vi "Auto Execute Commands.vi"() -> ()   [LabVIEW 2019]
uses:
  Controls/Auto Controls.ctl
  <vilib>/Rock Robotics/WPI/Solenoid/WPI_SolenoidValue.ctl
  <vilib>/Rock Robotics/WPI/Solenoid/WPI_SolenoidSetEnum.vi
panel:
  in  "Auto Commands":T1=[{"Drive Duration"=0.0, "Left Speed"=0.0, "Right Speed"=0.0, "Set Point"=0.0, "Set Point Duration"=0.0, "Command"=enum."Drive Forwards"}, {"Drive Duration"=0.0, "Left Speed"=0.0, "Right Speed"=0.0, "Set Point"=0.0, "Set Point Duration"=0.0, "Command"=enum."Drop Intake"}, {"Drive Duration"=0.0, "Left Speed"=0.0, "Right Speed"=0.0, "Set Point"=0.0, "Set Point Duration"=0.0, "Command"=enum."Drive Forwards"}, {"Drive Duration"=0.0, "Left Speed"=0.0, "Right Speed"=0.0, "Set Point"=0.0, "Set Point Duration"=0.0, "Command"=enum."Stop"}, {"Drive Duration"=0.0, "Left Speed"=0.0, "Right Speed"=0.0, "Set Point"=0.0, "Set Point Duration"=0.0, "Command"=enum."Intake"}, {"Drive Duration"=0.0, "Left Speed"=0.0, "Right Speed"=0.0, "Set Point"=0.0, "Set Point Duration"=0.0, "Command"=enum."Shooter"}, {"Drive Duration"=0.0, "Left Speed"=0.0, "Right Speed"=0.0, "Set Point"=0.0, "Set Point Duration"=0.0, "Command"=enum."Transfer"}]
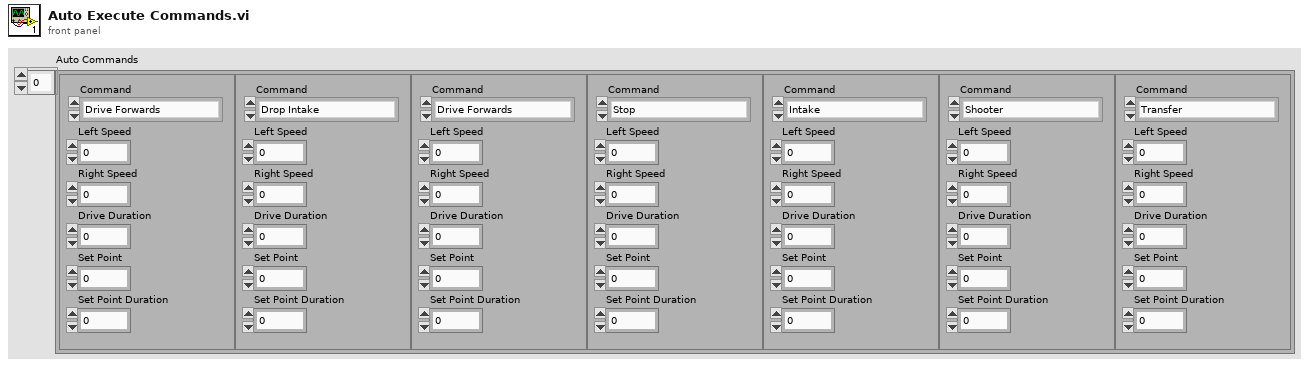
[diagram p1: front panel]
types:
  T1 = typedef "Auto Controls.ctl" = cluster{"Drive Duration":dbl, "Left Speed":dbl, "Right Speed":dbl, "Set Point":dbl, "Set Point Duration":dbl, "Command":enum16{"Drive Forwards", "Drive Backwards", "Stop", "Turn Left", "Turn Right", "Drop Intake", "Lift Intake", "Intake", "Shooter", "Transfer", "Wait"}}[]
  T2 = typedef "WPI_SolenoidValue.ctl" = enum16{"Off", "On", "Forward", "Reverse"}
  T3 = enum16{"Drive Forwards", "Drive Backwards", "Stop", "Turn Left", "Turn Right", "Drop Intake", "Lift Intake", "Intake", "Shooter", "Transfer", "Wait"}
  T4 = typedef "WPI_SolenoidDevRef.ctl" = cluster{"DevStatus":errorcluster, "Pneumatics Control Module":u8, "Forward Solenoid Channel":T5, "Reverse Solenoid Channel":T5}
  T5 = typedef "WPI_SolenoidChannel.ctl" = enum8{"Solenoid 0", "Solenoid 1", "Solenoid 2", "Solenoid 3", "Solenoid 4", "Solenoid 5", "Solenoid 6", "Solenoid 7", "Invalid"}
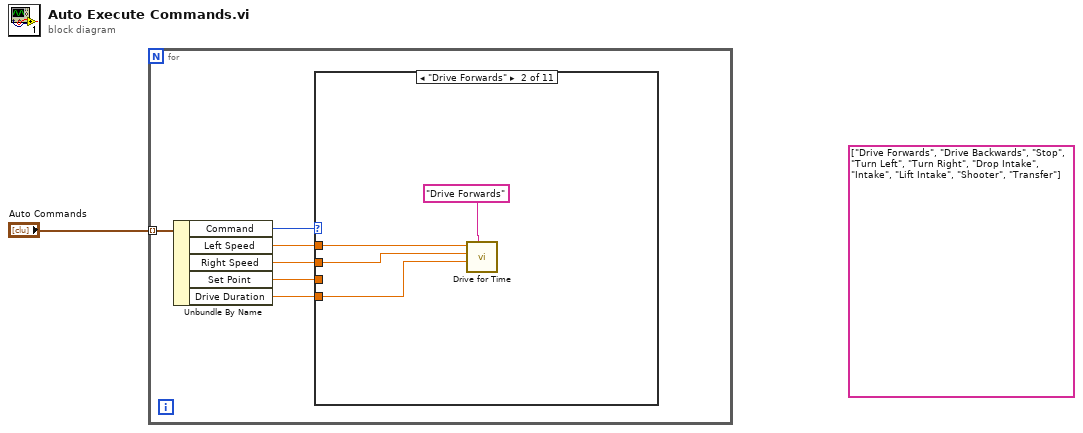
[diagram p0: block diagram]
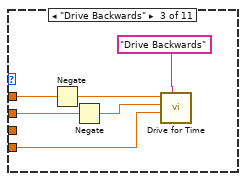
[diagram p3: hidden frame]
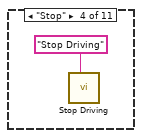
[diagram p4: hidden frame]
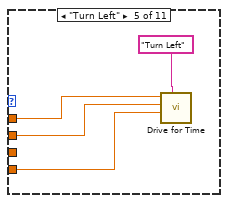
[diagram p5: hidden frame]
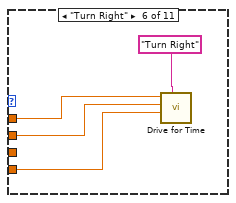
[diagram p6: hidden frame]
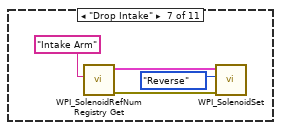
[diagram p7: hidden frame]
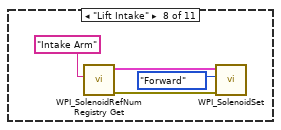
[diagram p8: hidden frame]
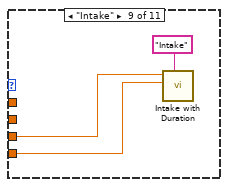
[diagram p9: hidden frame]
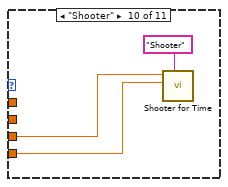
[diagram p10: hidden frame]
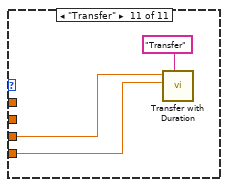
[diagram p11: hidden frame]
diagram:
  (unwired) string[] ["Drive Forwards", "Drive Backwards", "Stop", "Turn Left", "Turn Right", "Drop Intake", "Intake", "Lift Intake", "Shooter", "Transfer"]
  n1 = for {
    tunnel: "Auto Commands" -> [w7] mode=indexing
    n2 = Unbundle By Name(w7) -> ("Command"=w6:T3, "Left Speed"=w5:dbl, "Right Speed"=w4:dbl, "Set Point"=w2:dbl, "Drive Duration"=w3:dbl)
    n3 = case shown="\"Drive Forwards\"" w6 {
      tunnel: w5 -> [_ w10 w16 _ w21 w25 _ _ _ _ _]
      tunnel: w4 -> [_ w9 w15 _ w20 w24 _ _ _ _ _]
      tunnel: w3 -> [_ w8 w14 _ w19 w23 _ _ w35 w38 w41]
      tunnel: w2 -> [_ _ _ _ _ _ _ _ w36 w39 w42]
      frame Default {
      }
      frame "Drive Forwards" {
        n4 = call "Drive for Time.vi"("Description"="Drive Forwards", "Seconds"=w8, "Right Speed"=w9, "Left Speed"=w10) -> ()  [unwired: 7 in, 1 out]
      }
      frame "Drive Backwards" {
        n5 = Negate(x=w16) -> (-x=w13:dbl)
        n6 = Negate(x=w15) -> (-x=w12:dbl)
        n7 = call "Drive for Time.vi"("Description"="Drive Backwards", "Seconds"=w14, "Right Speed"=w12, "Left Speed"=w13) -> ()  [unwired: 7 in, 1 out]
      }
      frame "Stop" {
        n8 = call "Stop Driving.vi"("Description"="Stop Driving") -> ()  [unwired: 10 in, 1 out]
      }
      frame "Turn Left" {
        n9 = call "Drive for Time.vi"("Description"="Turn Left", "Seconds"=w19, "Right Speed"=w20, "Left Speed"=w21) -> ()  [unwired: 7 in, 1 out]
      }
      frame "Turn Right" {
        n10 = call "Drive for Time.vi"("Description"="Turn Right", "Seconds"=w23, "Right Speed"=w24, "Left Speed"=w25) -> ()  [unwired: 7 in, 1 out]
      }
      frame "Drop Intake" {
        n11 = call <vilib>:"WPI_SolenoidRefNum Registry Get.vi"("refnum name"="Intake Arm") -> ("error out"=w28:errorcluster, "SolenoidDevRef"=w29:T4)  [unwired: 9 in]
        n12 = call-poly <vilib>:"WPI_SolenoidSet.vi"("error in (no error)"=w28, "Value"=WPI_SolenoidValue."Reverse", "SolenoidDevRef"=w29) -> ()  [unwired: 7 in, 2 out]
      }
      frame "Lift Intake" {
        n13 = call <vilib>:"WPI_SolenoidRefNum Registry Get.vi"("refnum name"="Intake Arm") -> ("error out"=w32:errorcluster, "SolenoidDevRef"=w33:T4)  [unwired: 9 in]
        n14 = call-poly <vilib>:"WPI_SolenoidSet.vi"("error in (no error)"=w32, "Value"=WPI_SolenoidValue."Forward", "SolenoidDevRef"=w33) -> ()  [unwired: 7 in, 2 out]
      }
      frame "Intake" {
        n15 = call "Intake with Duration.vi"("Description"="Intake", "Duration (s)"=w35, "Setpoint"=w36) -> ()  [unwired: 8 in, 1 out]
      }
      frame "Shooter" {
        n16 = call "Shooter for Time.vi"("Description"="Shooter", "Duration (s)"=w38, "Setpoint"=w39) -> ()  [unwired: 8 in, 1 out]
      }
      frame "Transfer" {
        n17 = call "Transfer with Duration.vi"("Description"="Transfer", "Duration (s)"=w41, "Setpoint"=w42) -> ()  [unwired: 8 in, 1 out]
      }
    }
  }
